vi "Initialize InitCallback Acknowledgment User Event.vi"(8 "error in (no error)":errorcluster) -> (0 "error out":errorcluster, 2 "Init'd":refnum<user-event>, 3 "InitCallbackAck Registration":refnum<event-registration>)   [LabVIEW 2019, in "grpc-lvsupport.lvlib"]
uses:
  grpc-lvsupport.lvlib
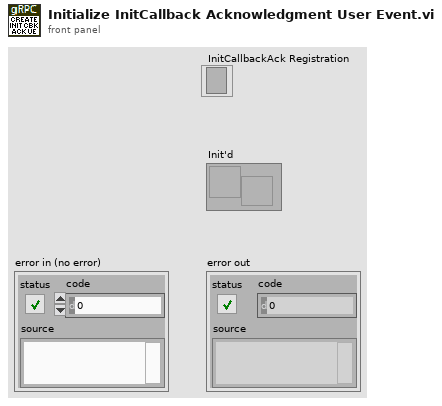
[diagram p1: front panel]
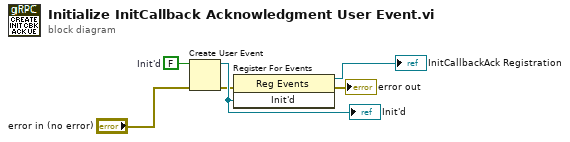
[diagram p0: block diagram]
diagram:
  w1 = FALSE  # Init'd
  n1 = Create User Event(user event datatype=w1, error in="error in (no error)") -> (user event=w3:refnum<user-event>, error out=w2:errorcluster)
  "Init'd" <- w3
  n2 = register-events(error in=w2, w3) -> (reference out=→"InitCallbackAck Registration":refnum<event-registration>, error out=→"error out":errorcluster)  [unwired: 1 in]
